vi "Get Plugin Address.vi"(8 "error in (no error)":errorcluster, 11 "CIF_UI in":refnum<class "CIF_UI.lvclass">) -> (0 "error out":errorcluster, 2 "Plugin Address":string, 3 "CIF_UI out":refnum<class "CIF_UI.lvclass">)   [LabVIEW 2021, in "CIF_UI.lvclass"]
uses:
  CIF_UI.lvclass
  CIF_UI.lvclass/CIF_UI.ctl
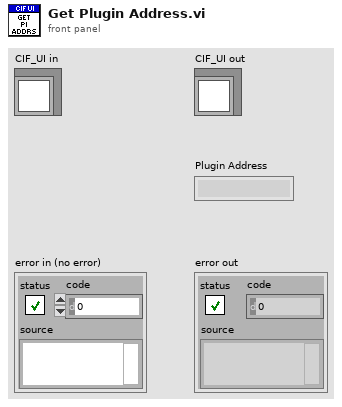
[diagram p1: front panel]
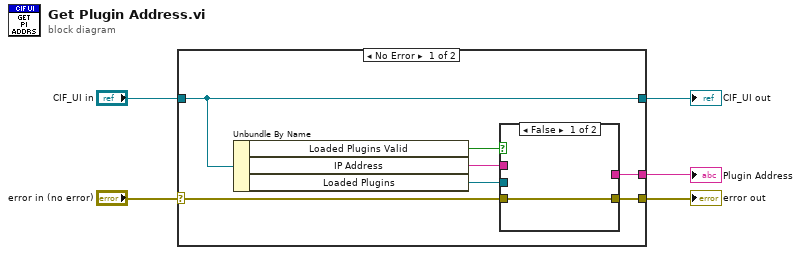
[diagram p0: block diagram]
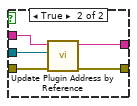
[diagram p2: hidden frame]
diagram:
  n1 = case shown="No Error" "error in (no error)" {
    selector: "error in (no error)" -> [w8 w20]
    tunnel: [w11 w20] -> w4
    tunnel: [w9 w19] -> w2
    tunnel: "CIF_UI in" -> [w9 w19]
    tunnel: [w10 _] -> w1
    frame No Error {
      n2 = Unbundle By Name(w9) -> ("Loaded Plugins Valid"=w6:bool, "IP Address"=w7:string, "Loaded Plugins"=w12:refnum<vi>)
      n3 = case shown="False" w6 {
        tunnel: w12 -> [_ w18]
        tunnel: [w13 w17] -> w11
        tunnel: [_ w16] -> w10
        tunnel: w8 -> [w13 w15]
        tunnel: w7 -> [_ w14]
        frame False {
        }
        frame True {
          n4 = call "Update Plugin Address by Reference.vi"("error in (no error)"=w15, "Loaded Plugins"=w18, "IP"=w14) -> ("error out"=w17:errorcluster, "Plugin Address"=w16:string)  [unwired: 7 in]
        }
      }
    }
    frame Error {
    }
  }
  "error out" <- w4
  "CIF_UI out" <- w2
  "Plugin Address" <- w1
